vi "Dashboard Main.vi"() -> ()   [LabVIEW 2012]
uses:
  <vilib>/Rock Robotics/WPI/Camera/WPI_CameraWhite Balance Values.ctl
  <vilib>/event_ctls.llb/eventvkey.ctl
  <vilib>/Utility/config.llb/Read Key (String).vi
  <vilib>/Utility/config.llb/Read Key (I32).vi
  <vilib>/Utility/config.llb/Write Key (String).vi
  <vilib>/Utility/config.llb/Write Key (I32).vi
  globals/Angle.vi
  <vilib>/Utility/config.llb/NI_LVConfig.lvlib
  AutonomousSelector.lvlib
  <vilib>/FTP/NI_FTP.lvlib
panel:
  in  "Tab Control":enum32{"Main", "Diagnostic"}(tab)
  in  "Viewer":enum32{"Camera", "Variables", "Files"}(tab)
  in  "Camera Settings":T1={"Frate Rate"=30, "Compression"=30, "Size"=1} {"Frate Rate" scale=1.0..30.0; "Size" items=["640x480", "320x240", "160x120"]}
  out "Mbps":dbl format="%#.1g"
  in  "DB Camera Config":bool
  out "Mbps":bool
  out "fps":dbl format="%#.1g"
  out "Image Error Message":string="Timeout in Camera Communications"
  out "Low Camera Image":T2(plugin-control) caption="Camera Image"
  out "High Camera Image":T2(plugin-control) caption="Camera Image"
  out "Tree":string(tree)
  in  "working directory":path=path "C:/BB/2013/Programming/Beachbot2013Dashboard"
  out "standard output":string
  in  "Transfer CSV to cRIO":bool
  in  "Transfer INI From cRIO":bool
  in  "Dashboard Tab":T3(tab)
  in  "LEDEnable":bool
  out "Battery Value":dbl(slide) scale=0.0..14.0 scale format="%#_2e"
  out "Battery":sgl(graph)
  out "Robot IP":string
  in  "Autonomous Mode":u16(ring)
  in  "Number":dbl caption="rightDriveP"
  in  "Preferences Tree":string(tree)
  in  "Save":bool
  in  "On/Off":bool caption="~S A V E~"
  in  "String":string caption="Strings"
  in  "Slider":dbl(slide) scale=0.0..100.0 scale format="%#_3g"
  in  "What is this?":bool
  in  "Test Name":u16(ring) items=["Select the test to run...", "Example Test", "-------------------------------", "List of tests is built in robot code.", "Replace with your own automated tests."]
  in  "Test Tree":string(tree)
  in  "Motor":cluster{"Value":dbl, "Enable":bool} {"Value" scale=-1.0..1.0 scale format="%#_3g"}
  out "Progress":T4 {"Test Progress" scale=0.0..100.0}
  in  "Rev/Fwd":cluster{"Forward":bool, "Reverse":bool}
  in  "Ring":u16(ring) items=["Auto", "Fixed indoor", "Fixed outdoor 1", "Fixed outdoor 2", "Fixed fluorescent 1", "Fixed fluorescent 2", "Hold current"]
  in  "Listbox":i32(listbox)
  out "Camera Image Diag":T2(plugin-control) caption="Camera Image"
  out "High Camera IP":string
  out "Low Camera IP":string
  out "Target Info":T5(array[cluster]) {"Center Position"."X" format="%#_3g"; "Center Position"."Y" format="%#_3g"}
  in  "Camera view angle":dbl[](array[numeric])=[48.0, 43.5]
  out "Processed Image":T2(plugin-control)
  in  "High Dilate_its":i32=5
  in  "High Erode_its":i32=5
  in  "High Brightness":i32=50
  in  "Low Dilate_its":i32=8
  in  "Low Erode_its":i32=7
  in  "Low Brightness":i32=50
  in  "Camera\nSelect H/L":bool=TRUE
  out "Mode":T6(ring)=enum."Auto Disabled"
  # "Robot IP:"
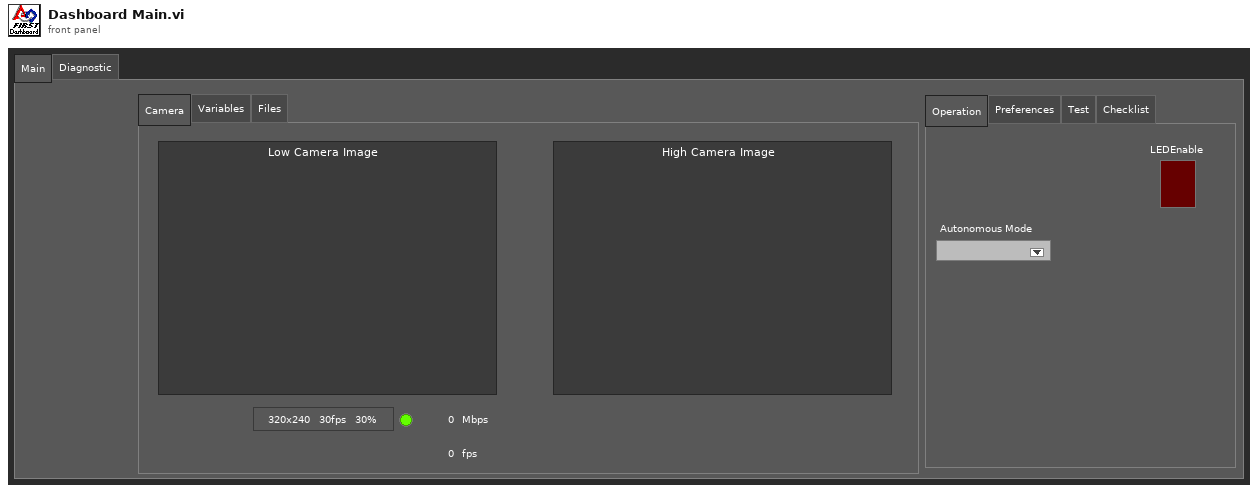
[diagram p1: front panel]
types:
  T1 = cluster{"Frate Rate":i32, "Compression":i32, "Size":u16}
  T2 = typedef "IMAQ Image.ctl" = refnum<image>
  T3 = enum32{"Operation", "Preferences", "Test", "Checklist"}
  T4 = cluster{"Test Progress":u8, "Test Progress Text":string}
  T5 = cluster{"Center Position":cluster{"X":dbl, "Y":dbl}, "Distance":dbl, "targetType":enum16{"Center", "Side", "Vertical"}}[]
  T6 = enum8{"Tele-Op Disabled", "Tele-Op Enabled", "Auto Disabled", "Auto Enabled", "Test Disabled", "Test Enabled", ""}
  T7 = typedef "Image Type" = u32
  T8 = typedef "WPI_CameraWhite Balance Values.ctl" = enum16{"Auto", "Fixed indoor", "Fixed outdoor 1", "Fixed outdoor 2", "Fixed fluorescent 1", "Fixed fluorescent 2", "Hold current"}
  T9 = typedef "SkeletonTrackState.ctl" = enum32{"NotTracked", "PositionOnly", "Tracked"}
  T10 = cluster{"TrackingState":u8[], "Position":cluster{"x":sgl, "y":sgl, "z":sgl}, cluster{"x":sgl, "y":sgl, "z":sgl, sgl}[], "TrackState":T9}
  T11 = cluster{cluster{"ScaledToPercentRange":dbl, "ScaledToPercentRange":dbl, "ScaledToPercentRange":dbl}, cluster{bool, bool, bool}}[]
  T12 = cluster{cluster{"ScaledToPercentRange":dbl, "ScaledToPercentRange":dbl, "ScaledToPercentRange":dbl}, cluster{bool, bool, bool}}
  T13 = typedef "LVRectTypeDef.ctl" = cluster{"Left":i16, "Top":i16, "Right":i16, "Bottom":i16}
  T14 = cluster{"Competition mode":bool, "Robot Link":bool, "Autonomous":bool, "Enabled":bool, "E-Stop":bool, "Simulated":bool, "TestMode":bool, "Docked Window":bool}
  T15 = typedef "NI_LVConfig.lvlib/Config Data RefNum.ctl" = refnum<k1>
  T16 = typedef "WPI_CameraDevRef.ctl" = cluster{"Camera Address":string, "CameraStatus":errorcluster, "Acquire Image Notifier":refnum<notifier>}
  T17 = typedef "eventvkey.ctl" = enum16{"ASCII", "Enter", "Return", "Shift", "Ctrl", "Alt", "Cmd", "Opt", "Caps", "NumLock", "Clear", "Break", "Up", "Down", "Left", "Right", "Insert", "Delete", "Home", "End", "PageUp", "PageDown", "Escape", "Help", "Pause", "ScrollLock", "F1", "F2", "F3", "F4", "F5", "F6", "F7", "F8", "F9", "F10", "F11", "F12", "F13", "F14", "F15", "F16", "F17", "F18", "F19", "F20", "F21", "F22", "F23", "F24", "Play", "VolumeUp", "VolumeDown", "Mute", "Two Byte Char"}
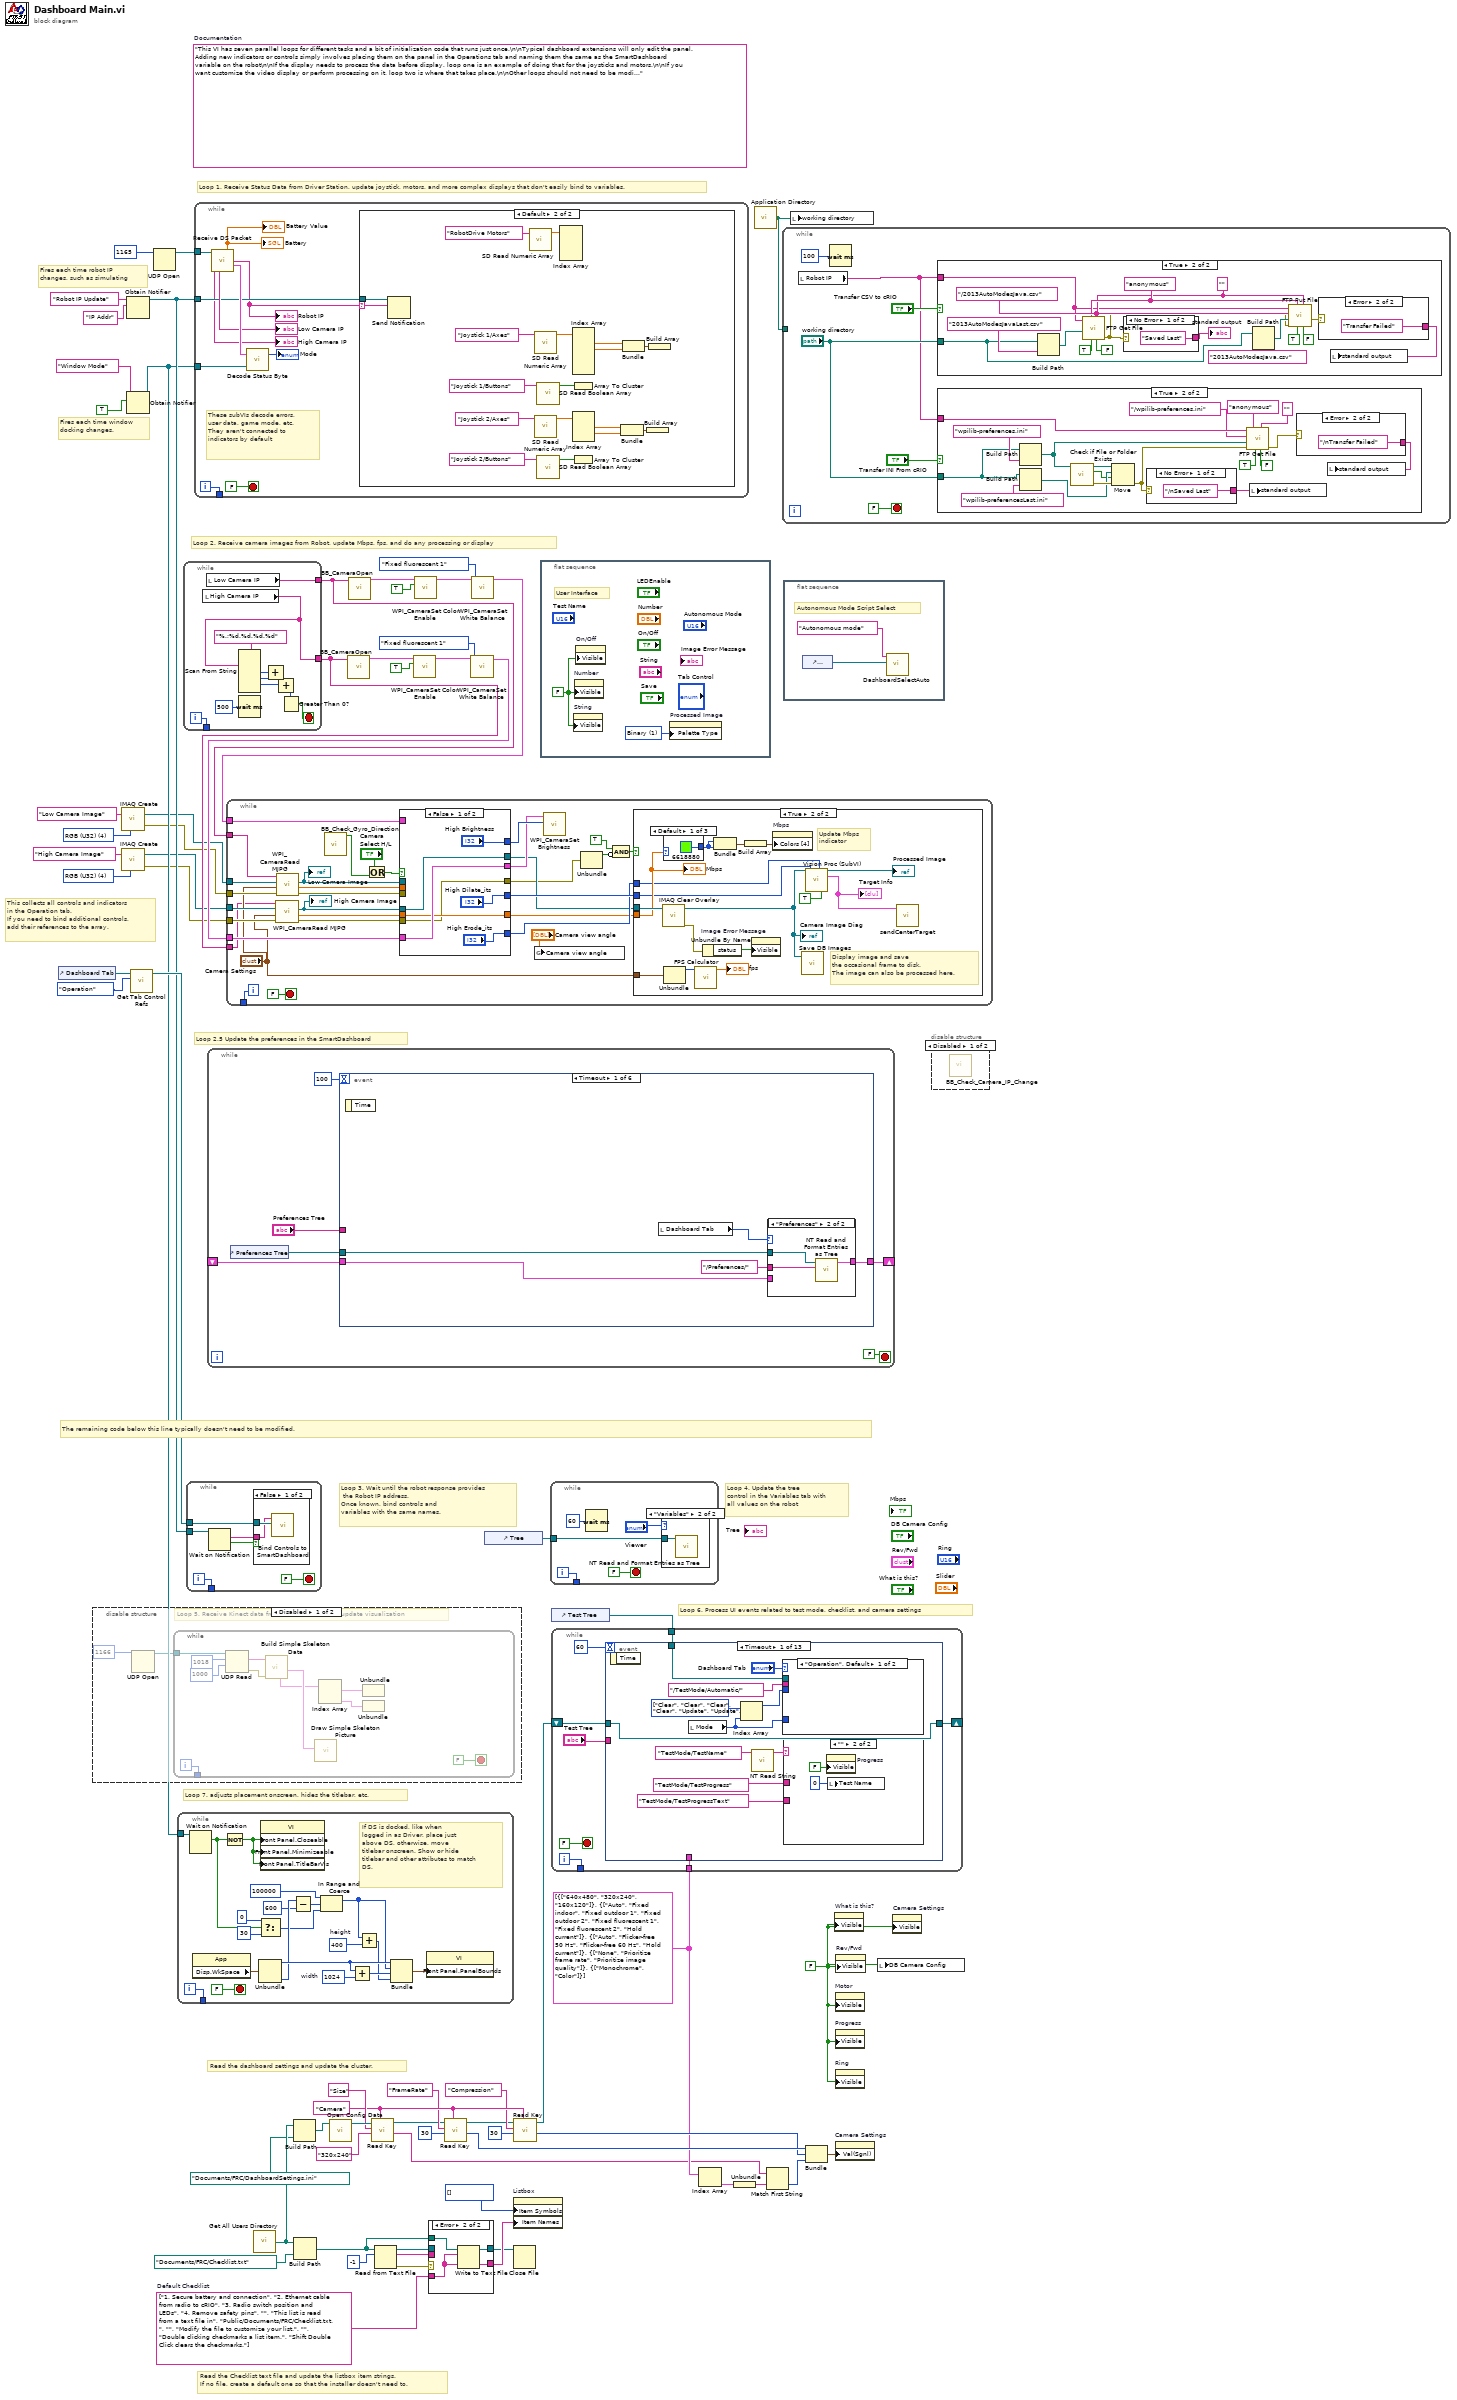
[diagram p0: block diagram]
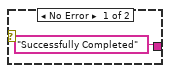
[diagram p3: hidden frame]
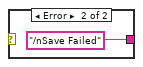
[diagram p4: hidden frame]
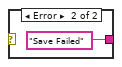
[diagram p6: hidden frame]
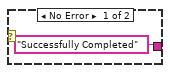
[diagram p7: hidden frame]
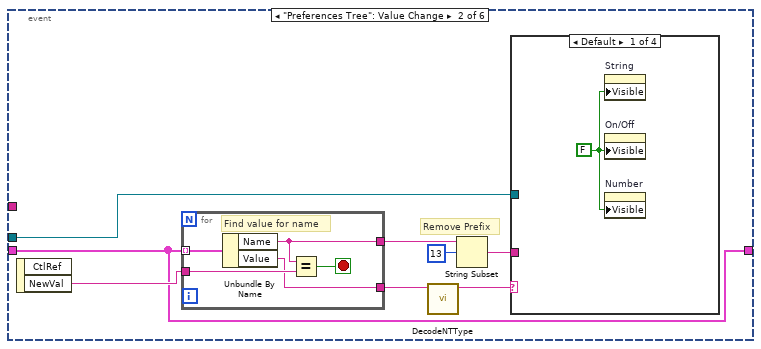
[diagram p10: hidden frame]
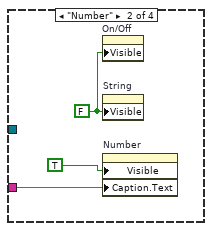
[diagram p11: hidden frame]
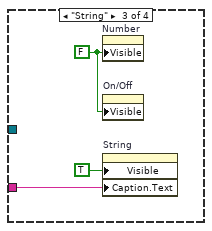
[diagram p12: hidden frame]
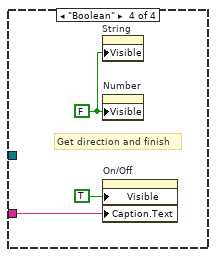
[diagram p13: hidden frame]
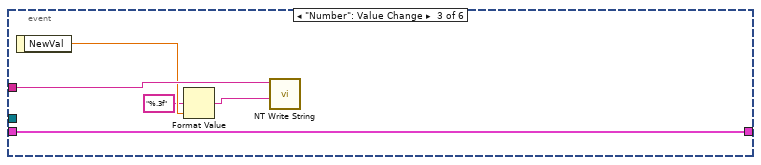
[diagram p14: hidden frame]
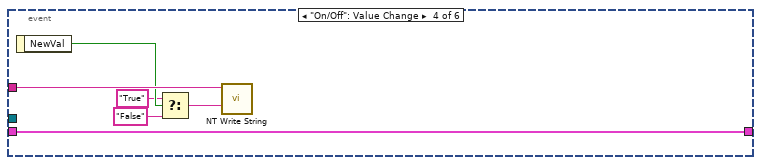
[diagram p15: hidden frame]
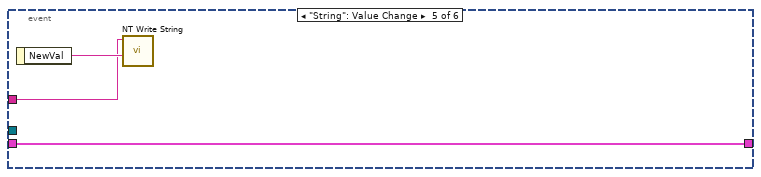
[diagram p16: hidden frame]
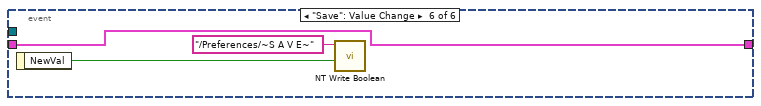
[diagram p17: hidden frame]
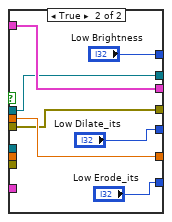
[diagram p20: hidden frame]
diagram:
  w7 = T7 4 items=["Grayscale (U8)", "Grayscale (I16)", "Grayscale (SGL)", "Complex (CSG)", "RGB (U32)", "HSL (U32)", "RGB (U64)"] ("Image Type")
  w8 = T7 4 items=["Grayscale (U8)", "Grayscale (I16)", "Grayscale (SGL)", "Complex (CSG)", "RGB (U32)", "HSL (U32)", "RGB (U64)"] ("Image Type")
  w42 = "Camera"
  w34 = cluster{string[]}[] [{["640x480", "320x240", "160x120"]}, {["Auto", "Fixed indoor", "Fixed outdoor 1", "Fixed outdoor 2", "Fixed fluorescent 1", "Fixed fluorescent 2", "Hold current"]}, {["Auto", "Flicker-free 50 Hz", "Flicker-free 60 Hz", "Hold current"]}, {["None", "Prioritize frame rate", "Prioritize image quality"]}, {["Monochrome", "Color"]}]
  w50 = string[] ["1. Secure battery and connection", "2. Ethernet cable from radio to cRIO", "3. Radio switch position and LEDs", "4. Remove safety pins", "", "This list is read from a text file in", "Public/Documents/FRC/Checklist.txt.", "", "Modify the file to customize your list.", "", "Double clicking checkmarks a list item.", "Shift Double Click clears the checkmarks."]  # Default Checklist
  w48 = FALSE ("Visible")
  (unwired) "This VI has seven parallel loops for different tasks and a bit of initialization code that runs just once.\n\nTypical dashboard extensions will only edit the panel. Adding new indicators or controls simply involves placing them on the panel in the Operations tab and naming them the same as the SmartDashboard variable on the robot\n\nIf the display needs to process the data before display, loop one is an example of doing that for the joysticks and motors.\n\nIf you want customize the video display or perform processing on it, loop two is where that takes place.\n\nOther loops should not need to be modified. They are pretty standard, and document the task they perform."  # Documentation
  # "Loop 2.5 Update the preferences in the SmartDashboard"
  # "Fires each time robot IP\nchanges, such as simulating"
  # "Fires each time window\ndocking changes."
  # "Read the Checklist text file and update the listbox item strings.\nIf no file, create a default one so that the installer doesn't need to."
  # "This collects all controls and indicators\nin the Operation tab.\nIf you need to bind additional controls,\nadd their references to the array."
  # "The remaining code below this line typically doesn't need to be modified."
  # "Loop 6. Process UI events related to test mode, checklist, and camera settings"
  # "Read the dashboard settings and update the cluster."
  # "Loop 4. Update the tree\ncontrol in the Variables tab with\nall values on the robot"
  # "Loop 3. Wait until the robot response provides\n the Robot IP address.\nOnce known, bind controls and\nvariables with the same names."
  # "Loop 7. adjusts placement onscreen, hides the titlebar, etc."
  # "Loop 1. Receive Status Data from Driver Station, update joystick, motors, and more complex displays that don't easily bind to variables."
  # "Loop 2. Receive camera images from Robot, update Mbps, fps, and do any processing or display"
  n1 = control-ref of="Dashboard Tab"() -> (w64:refnum<vi>)
  n2 = disable-structure shown="Disabled" {
    frame Disabled {
      # "Loop 5. Receive Kinect data from Driver Station and update visualization"
      n3 = UDP Open(11:u16 1166 ("port")) -> (port=w68:refnum<k16>)  [unwired: 2 in, 4 out]
      n4 = while {
        tunnel: w68 -> [w78]
        tunnel: [w71] -> _
        i -> [w71]
        stop <- FALSE stop-if-true
        n5 = UDP Read(connection ID=w78, max size (548)=1018 ("bytes to read"), timeout ms (25000)=1000) -> (data out=w76:string, error out=w70:errorcluster)  [unwired: 1 in, 3 out]
        n6 = call "Build Simple Skeleton Data.vi"("error in (no error)"=w70, "data in"=w76) -> ("Skeleton Data"=w77:T10, "Simple Joystick Info"=w74:T11)  [unwired: 5 in, 3 out]
        n7 = call "Draw Simple Skeleton Picture.vi"("Simple Skeleton"=w77) -> ()  [unwired: 10 in, 1 out]
        n8 = Index Array(array=w74) -> (element #1=w73:T12, element #2=w72:T12)  [unwired: 2 in]
        n9 = Unbundle(w73) -> ()  [unwired: 2 out]
        n10 = Unbundle(w72) -> ()  [unwired: 2 out]
      }
    }
    frame Enabled {
    }
  }
  n11 = call "IMAQ Create"("Image Name"="Low Camera Image", "Image Type"=w7) -> ("New Image"=w2:T2, "error out"=w3:errorcluster)  [unwired: 2 in, 1 out]
  n12 = call "IMAQ Create"("Image Name"="High Camera Image", "Image Type"=w8) -> ("New Image"=w4:T2, "error out"=w5:errorcluster)  [unwired: 2 in, 1 out]
  n13 = Obtain Notifier(name (unnamed)="Robot IP Update", notification data type="IP Addr" ("name (unnamed)")) -> (notifier out=w61:refnum<notifier>)  [unwired: 2 in, 2 out]
  n14 = Obtain Notifier(name (unnamed)="Window Mode", notification data type=TRUE) -> (notifier out=w54:refnum<notifier>)  [unwired: 2 in, 2 out]
  n15 = call <vilib>:"Get Tab Control Refs.vi"("Page Index"=enum32{"Operation", "Test"}."Operation" ("Dashboard Tab"), "TabControl in"=w64) -> ("ControlsOnPage"=w65:refnum<vi>[])  [unwired: 9 in]
  n16 = UDP Open(11:u16 1165 ("port")) -> (port=w66:refnum<k16>)  [unwired: 2 in, 4 out]
  n17 = while {
    tunnel: w54 -> [w99]
    tunnel: [w97] -> _
    i -> [w97]
    stop <- FALSE stop-if-true
    w89 = 1024  # width
    w92 = 400  # height
    # "If DS is docked, like when\nlogged in as Driver, place just\nabove DS, otherwise, move\ntitlebar onscreen. Show or hide\ntitlebar and other attributes to match\nDS."
    n18 = Wait on Notification(notifier=w99) -> (notification=w84:bool)  [unwired: 3 in, 3 out]
    n19 = property class="App"() -> ("Disp.WkSpace"=w95:T13)  [unwired: 2 in, 2 out]
    n20 = Not(x=w84) -> (.not. x?=w98:bool)
    n21 = Unbundle(w95) -> ("Left"=w93:i16, "Bottom"=w90:i16)  [unwired: 2 out]
    n22 = Select(t=0, s=w84, f=30) -> (s? t:f=w83:i32)
    n23 = property class="VI"("Front Panel.Closeable"=w98, "Front Panel.Minimizeable"=w98, "Front Panel.TitleBarVis"=w98) -> ()  [unwired: 2 in, 2 out]
    n24 = Subtract(x=w90, y=600) -> (x-y=w87:i32)
    n25 = In Range and Coerce(upper limit=100000, x=w87, lower limit=w83) -> (coerced(x)=w81:i32)  [unwired: 1 out]
    n26 = Add(x=w93, y=w89) -> (x+y=w94:i32)
    n27 = Add(x=w81, y=w92) -> (x+y=w91:i32)
    n28 = Bundle("Left"=w93, w81, w94, w91) -> (w96:cluster{"Left":i16, i32, i32, i32})  [unwired: 1 out]
    n29 = property class="VI"("Front Panel.PanelBounds"=w96) -> ()  [unwired: 2 in, 2 out]
  }
  n30 = while {
    tunnel: [w111] -> w11
    tunnel: [w104] -> w10
    tunnel: [w102] -> _
    i -> [w102]
    stop <- w103 stop-if-true
    n31 = local read "High Camera IP"() -> (w104:string)
    n32 = local read "Low Camera IP"() -> (w111:string)
    n33 = Scan From String(format string="%.;%d.%d.%d.%d", input string=w104) -> (output 1=w108:i32, output 2=w109:i32, output 3=w106:i32)  [unwired: 2 in, 8 out]
    n34 = Wait (ms)(milliseconds to wait=u32 500) -> ()  [unwired: 1 out]
    n35 = Add(x=w108, y=w109) -> (x+y=w107:i32)
    n36 = Add(x=w107, y=w106) -> (x+y=w105:i32)
    n37 = Greater Than 0?(x=w105) -> (x > 0?=w103:bool)
  }
  n38 = while {
    tunnel: w65 -> [w117]
    tunnel: w61 -> [w114]
    tunnel: [w112] -> _
    i -> [w112]
    stop <- FALSE stop-if-true
    n39 = Wait on Notification(notifier=w114) -> (notification=w113:string, timed out?=w115:bool)  [unwired: 3 in, 2 out]
    n40 = case shown="False" w115 {
      tunnel: w117 -> [w119 _]
      tunnel: w113 -> [w118 _]
      frame False {
        n41 = call <vilib>:"Bind Controls to SmartDashboard.vi"("Bound Control Refs"=w119, "Server IP Address"=w118) -> ()  [unwired: 10 in]
      }
      frame True {
      }
    }
  }
  n42 = while {
    tunnel: w66 -> [w128]
    tunnel: w61 -> [w122]
    tunnel: w54 -> [w126]
    tunnel: [w123] -> _
    i -> [w123]
    stop <- FALSE stop-if-true
    # "These subVIs decode errors, user data, game mode, etc.\nThey aren't connected to indicators by default"
    n43 = call "Receive DS Packet.vi"("Recv Socket"=w128) -> ("Battery"=→"Battery" →"Battery Value":sgl, "Robot IP Address"=w121:string, "Status"=w129:T14, "High Camera IP Address"=→"High Camera IP":string, "Low Camera IP Address"=→"Low Camera IP":string)  [unwired: 1 in, 9 out]
    "Robot IP" <- w121
    n44 = call "Decode Status Byte.vi"("Window Mode Notifier"=w126, "Status"=w129) -> ("Mode"=→"Mode":T6)  [unwired: 1 out]
    n45 = case shown="Default" w121 {
      selector: w121 -> [_ w131]
      tunnel: w122 -> [_ w132]
      frame "0.0.0.0" {
        # "Robot not responding, don't poll the variables"
      }
      frame Default {
        n46 = Send Notification(notification=w131, notifier=w132) -> ()  [unwired: 1 in, 2 out]
        n47 = call <vilib>:"SD Read Numeric Array.vi"("Name"="RobotDrive Motors") -> ("Numeric Array"=w145:dbl[])  [unwired: 8 in, 2 out]
        n48 = call <vilib>:"SD Read Numeric Array.vi"("Name"="Joystick 1/Axes") -> ("Numeric Array"=w143:dbl[])  [unwired: 8 in, 2 out]
        n49 = call <vilib>:"SD Read Numeric Array.vi"("Name"="Joystick 2/Axes") -> ("Numeric Array"=w139:dbl[])  [unwired: 8 in, 2 out]
        n50 = call <vilib>:"SD Read Boolean Array.vi"("Name"="Joystick 1/Buttons") -> ("Boolean Array"=w144:bool[])  [unwired: 8 in, 2 out]
        n51 = call <vilib>:"SD Read Boolean Array.vi"("Name"="Joystick 2/Buttons") -> ("Boolean Array"=w138:bool[])  [unwired: 8 in, 2 out]
        n52 = Index Array(array=w145) -> ()  [unwired: 4 in, 4 out]
        n53 = Array To Cluster(array=w144) -> ()  [unwired: 1 out]
        n54 = Array To Cluster(array=w138) -> ()  [unwired: 1 out]
        n55 = Index Array(array=w143) -> (element #1=w141:dbl, element #2=w142:dbl)  [unwired: 6 in, 4 out]
        n56 = Index Array(array=w139) -> (element #1=w134:dbl, element #2=w133:dbl)  [unwired: 3 in, 1 out]
        n57 = Bundle("Numeric"=w134, "Numeric"=w133) -> (w135:cluster{"Numeric":dbl, "Numeric":dbl})  [unwired: 1 in]
        n58 = Bundle("Numeric"=w141, "Numeric"=w142) -> (w140:cluster{"Numeric":dbl, "Numeric":dbl})  [unwired: 1 in]
        n59 = Build Array(w135) -> ()  [unwired: 1 out]
        n60 = Build Array(w140) -> ()  [unwired: 1 out]
      }
    }
  }
  n61 = while {
    shift-right: [w150] -> _
    shift-left: _ -> [w149]
    stop <- FALSE stop-if-true
    n62 = control-ref of="Preferences Tree"() -> (w152:refnum<vi>)
    n63 = event shown="[0] Timeout" {
      selector: _ -> [_ _ _ _ _ _]
      dyn-events: _ -> [_ _ _ _ _ _]
      timeout: u32 100 ("milliseconds to wait") -> [_ _ _ _ _ _]
      tunnel: w152 -> [w157 w170 _ _ _ _]
      tunnel: "Preferences Tree" -> [_ _ w191 w197 w199 _]
      tunnel: [w158 w164 w190 w196 w198 w201] -> w150
      tunnel: w149 -> [w156 w164 w190 w196 w198 w201]
      event Timeout {
        n64 = event-data() -> ()  [unwired: 1 in, 1 out]
        n65 = local read "Dashboard Tab"() -> (w155:T3)
        n66 = case shown="\"Preferences\"" w155 {
          tunnel: w157 -> [_ w163]
          tunnel: "/Preferences/" ("Name Pattern") -> [_ w162]
          tunnel: [w160 w161] -> w158
          tunnel: w156 -> [w160 _]
          frame "Operation", Default {
          }
          frame "Preferences" {
            n67 = call <vilib>:"NT Read and Format Entries as Tree.vi"("Name Pattern"=w162, "Tree Refnum"=w163) -> ("Formatted Strings"=w161:cluster{"Name":string, "Value":string}[])  [unwired: 8 in, 1 out]
          }
        }
      }
      event "Preferences Tree": Value Change {
        # "Remove Prefix"
        n68 = event-data() -> ("NewVal"=w168:string)  [unwired: 1 in, 1 out]
        n69 = for {
          tunnel: w164 -> [w176] mode=indexing
          tunnel: w168 -> [w175]
          tunnel: [w173] -> w169
          tunnel: [w172] -> w167
          stop <- w174 stop-if-true
          # "Find value for name"
          n70 = Unbundle By Name(w176) -> ("Name"=w172:string, "Value"=w173:string)
          n71 = Equal?(x=w172, y=w175) -> (x = y?=w174:bool)
        }
        n72 = call "DecodeNTType.vi"("string"=w169) -> ("type"=w171:string)  [unwired: 7 in, 3 out]
        n73 = String Subset(string=w167, offset (0)=13) -> (substring=w166:string)  [unwired: 1 in]
        n74 = case shown="Default" w171 {
          tunnel: w170 -> [_ _ _ _]
          tunnel: w166 -> [_ w178 w181 w185]
          frame Default {
            w177 = FALSE ("Visible")
            n75 = property on="String" class="Str"("Visible"=w177) -> ()  [unwired: 2 in, 2 out]
            n76 = property on="On/Off" class="Bool (strict)"("Visible"=w177) -> ()  [unwired: 2 in, 2 out]
            n77 = property on="Number" class="DigNum (strict)"("Visible"=w177) -> ()  [unwired: 2 in, 2 out]
          }
          frame "Number" {
            w179 = FALSE ("Visible")
            n78 = property on="On/Off" class="Bool (strict)"("Visible"=w179) -> ()  [unwired: 2 in, 2 out]
            n79 = property on="String" class="Str"("Visible"=w179) -> ()  [unwired: 2 in, 2 out]
            n80 = property on="Number" class="DigNum (strict)"("Visible"=TRUE, "Caption.Text"=w178) -> ()  [unwired: 2 in, 2 out]
          }
          frame "String" {
            w182 = FALSE ("Visible")
            n81 = property on="Number" class="DigNum (strict)"("Visible"=w182) -> ()  [unwired: 2 in, 2 out]
            n82 = property on="On/Off" class="Bool (strict)"("Visible"=w182) -> ()  [unwired: 2 in, 2 out]
            n83 = property on="String" class="Str"("Visible"=TRUE, "Caption.Text"=w181) -> ()  [unwired: 2 in, 2 out]
          }
          frame "Boolean" {
            w184 = FALSE ("Visible")
            # "Get direction and finish"
            n84 = property on="String" class="Str"("Visible"=w184) -> ()  [unwired: 2 in, 2 out]
            n85 = property on="Number" class="DigNum (strict)"("Visible"=w184) -> ()  [unwired: 2 in, 2 out]
            n86 = property on="On/Off" class="Bool (strict)"("Visible"=TRUE, "Caption.Text"=w185) -> ()  [unwired: 2 in, 2 out]
          }
        }
      }
      event "Number": Value Change {
        n87 = event-data() -> ("NewVal"=w189:dbl)  [unwired: 1 in]
        n88 = Format Value(format string="%.3f", value (0)=w189) -> (output string=w187:string)  [unwired: 1 in]
        n89 = call <vilib>:"NT Write String.vi"("String"=w187, "Name"=w191) -> ()  [unwired: 9 in, 1 out]
      }
      event "On/Off": Value Change {
        n90 = event-data() -> ("NewVal"=w195:bool)  [unwired: 1 in]
        n91 = Select(t="True", s=w195, f="False") -> (s? t:f=w192:string)
        n92 = call <vilib>:"NT Write String.vi"("String"=w192, "Name"=w197) -> ()  [unwired: 9 in, 1 out]
      }
      event "String": Value Change {
        n93 = event-data() -> ("NewVal"=w200:string)  [unwired: 1 in]
        n94 = call <vilib>:"NT Write String.vi"("String"=w200, "Name"=w199) -> ()  [unwired: 9 in, 1 out]
      }
      event "Save": Value Change {
        n95 = event-data() -> ("NewVal"=w203:bool)  [unwired: 1 in]
        n96 = call <vilib>:"NT Write Boolean.vi"("Boolean"=w203, "Name"="/Preferences/~S A V E~") -> ()  [unwired: 9 in, 1 out]
      }
    }
  }
  n97 = call "Get All Users Directory.vi"() -> ("All User Path"=w47:path)
  n98 = Build Path(base path=w47, name or relative path=path "Documents/FRC/DashboardSettings.ini") -> (appended path=w46:path)
  n99 = Build Path(base path=w47, name or relative path=path "Documents/FRC/Checklist.txt") -> (appended path=w51:path)
  n100 = call <vilib>:"Open Config Data.vi"("configuration file path"=w46) -> ("refnum"=w45:T15)  [unwired: 8 in, 2 out]
  n101 = call "BB_CameraOpen.vi"("Camera Address"=w10) -> ("CameraDevRef"=w17:T16)  [unwired: 9 in, 1 out]
  n102 = call "BB_CameraOpen.vi"("Camera Address"=w11) -> ("CameraDevRef"=w21:T16)  [unwired: 9 in, 1 out]
  n103 = call-poly <vilib>:"Read Key.vi"("section"=w42, "default value"="320x240", "key"="Size", "refnum"=w45) -> ("value"=w32:string, "refnum out"=w27:T15)  [unwired: 2 in, 4 out]
  n104 = Read from Text File(file (use dialog)=w51, count=-1 ("timeout ms (25000)")) -> (refnum out=w29:refnum<file>, text=w52:string[], error out=w53:errorcluster)  [unwired: 2 in, 1 out]
  n105 = call <vilib>:"WPI_CameraSet Color Enable.vi"("Color Enabled"=TRUE, "CameraDevRef"=w17) -> ("CameraDevRef Out"=w15:T16)  [unwired: 8 in, 1 out]
  n106 = call <vilib>:"WPI_CameraSet Color Enable.vi"("Color Enabled"=TRUE, "CameraDevRef"=w21) -> ("CameraDevRef Out"=w19:T16)  [unwired: 8 in, 1 out]
  n107 = case shown="Error" w53 {
    tunnel: w52 -> [w205 _]
    tunnel: [w205 w207] -> w49
    tunnel: w50 -> [_ w207]
    tunnel: w51 -> [_ w208]
    tunnel: [w204 w206] -> w28
    tunnel: w29 -> [w204 _]
    frame No Error {
    }
    frame Error {
      n108 = Write to Text File(file (use dialog)=w208, text=w207) -> (refnum out=w206:refnum<file>)  [unwired: 2 in, 2 out]
    }
  }
  n109 = call-poly <vilib>:"Read Key.vi"("section"=w42, "default value"=30, "key"="FrameRate", "refnum"=w27) -> ("value"=w37:i32, "refnum out"=w26:T15)  [unwired: 1 in, 5 out]
  n110 = call <vilib>:"WPI_CameraSet White Balance.vi"("White Balance"=WPI_CameraWhite_Balance_Values."Fixed fluorescent 1", "CameraDevRef"=w15) -> ("CameraDevRef Out"=w13:T16)  [unwired: 8 in, 1 out]
  n111 = call <vilib>:"WPI_CameraSet White Balance.vi"("White Balance"=WPI_CameraWhite_Balance_Values."Fixed fluorescent 1", "CameraDevRef"=w19) -> ("CameraDevRef Out"=w12:T16)  [unwired: 8 in, 1 out]
  n112 = while {
    tunnel: [w238] -> _
    tunnel: w13 -> [w230]
    tunnel: w12 -> [w231]
    tunnel: w10 -> [w212]
    tunnel: w11 -> [w213]
    tunnel: w5 -> [w224]
    tunnel: w4 -> [w223]
    tunnel: w3 -> [w222]
    tunnel: w2 -> [w220]
    i -> [w238]
    stop <- FALSE stop-if-true
    n113 = call <vilib>:"WPI_CameraRead MJPG.vi"("error in"=w224, "Camera Settings"="Camera Settings", "Image"=w223, "address"=w212) -> ("error out"=w216:errorcluster, "Bandwidth (kbps)"=w215:dbl, "Image Out"=w214:T2)  [unwired: 5 in]
    "High Camera Image" <- w214
    n114 = call <vilib>:"WPI_CameraRead MJPG.vi"("error in"=w222, "Camera Settings"="Camera Settings", "Image"=w220, "address"=w213) -> ("error out"=w218:errorcluster, "Bandwidth (kbps)"=w219:dbl, "Image Out"=w217:T2)  [unwired: 5 in]
    "Low Camera Image" <- w217
    n115 = call "BB_Check_Gyro_Direction.vi"() -> ("chgDirection"=w226:bool)  [unwired: 11 in]
    n116 = Or(x="Camera\nSelect H/L", y=w226) -> (x .or. y?=w227:bool)
    n117 = case shown="False" w227 {
      tunnel: w231 -> [_ w253]
      tunnel: [w243 w253] -> w229
      tunnel: ["High Dilate_its" "Low Dilate_its"] -> w233
      tunnel: ["High Erode_its" "Low Erode_its"] -> w232
      tunnel: ["High Brightness" "Low Brightness"] -> w234
      tunnel: w230 -> [w243 _]
      tunnel: [w242 w249] -> w210
      tunnel: w219 -> [_ w248]
      tunnel: w218 -> [_ w247]
      tunnel: w217 -> [_ w249]
      tunnel: w216 -> [w240 _]
      tunnel: w215 -> [w241 _]
      tunnel: w214 -> [w242 _]
      tunnel: [w241 w248] -> w211
      tunnel: [w240 w247] -> w209
      frame False {
      }
      frame True {
      }
    }
    n118 = global write "Angle.vi" "Camera view angle"("Camera view angle") -> ()
    n119 = call <vilib>:"WPI_CameraSet Brightness.vi"("Brightness"=w234, "CameraDevRef"=w229) -> ()  [unwired: 8 in, 2 out]
    n120 = Unbundle(w209) -> ("status"=w237:bool)  [unwired: 2 out]
    n121 = Compound Arithmetic op=AND(TRUE, invert w237) -> (w236:bool)
    n122 = case shown="True" w236 {
      tunnel: "Camera Settings" -> [_ w262]
      tunnel: w210 -> [_ w265]
      tunnel: w211 -> [_ w264]
      tunnel: w233 -> [_ w259]
      tunnel: w232 -> [_ w258]
      frame False {
        # "Sleep for 500ms"
        n123 = Wait Until Next ms Multiple(millisecond multiple=u32 500) -> ()  [unwired: 1 out]
      }
      frame True {
        # "Display image and save\nthe occasional frame to disk.\nThe image can also be processed here."
        # "Update Mbps\nindicator"
        n124 = call "IMAQ Clear Overlay"("Image"=w265) -> ("error out"=w269:errorcluster, "Image Out"=w257:T2)  [unwired: 2 in, 7 out]
        "Camera Image Diag" <- w257
        n125 = case shown="Default" w264 {
          tunnel: [u32 6618880 ("Color Box") u32 16776722 ("Color Box") u32 16716800 ("Color Box")] -> w266
          frame Default {
          }
          frame 4, 5 {
          }
          frame 6.. {
          }
        }
        n126 = Unbundle(w262) -> ("Frate Rate"=w261:i32)  [unwired: 2 out]
        n127 = call "FPS Calculator.vi"("Average Count"=w261) -> ("fps"=→"fps":dbl)  [unwired: 10 in]
        n128 = Unbundle By Name(w269) -> ("status"=w270:bool)
        n129 = Bundle("Color Box"=w266, "Color Box"=w266) -> (w268:cluster{"Color Box":u32, "Color Box":u32})  [unwired: 1 out]
        n130 = Build Array(w268) -> (w267:cluster{"Color Box":u32, "Color Box":u32}[])
        n131 = property on="Image Error Message" class="Str"("Visible"=w270) -> ()  [unwired: 2 in, 2 out]
        n132 = property on="Mbps" class="Bool (strict)"("Colors [4]"=w267) -> ()  [unwired: 2 in, 2 out]
        n133 = call "Save DB Images.vi"("Image"=w257) -> ()  [unwired: 2 in, 1 out]
        n134 = call "Vision Proc (SubVI).vi"("Image In"=w257, "Dilate_its"=w259, "Erode_its"=w258, "Annotate"=TRUE) -> ("Processed Image"=→"Processed Image":T2, "Target Info"=w255:T5)  [unwired: 19 in, 3 out]
        "Target Info" <- w255
        n135 = call "sendCenterTarget.vi"("Target Info"=w255) -> ()  [unwired: 11 in]
        "Mbps" <- w264
      }
    }
  }
  n136 = control-ref of="Tree"() -> (w23:refnum<vi>)
  n137 = property on="Listbox" class="LstBox (strict)"("Item Symbols"=i32[] [], "Item Names"=w49) -> ()  [unwired: 2 in, 2 out]
  n138 = Close File(refnum=w28) -> ()  [unwired: 1 in, 2 out]
  n139 = call-poly <vilib>:"Read Key.vi"("section"=w42, "default value"=30, "key"="Compression", "refnum"=w26) -> ("value"=w36:i32, "refnum out"=w24:T15)  [unwired: 1 in, 5 out]
  n140 = flat-sequence {
    frame #0 {
      w274 = FALSE ("Visible")
      w275 = u32 1 items=["Grayscale", "Binary", "Gradient", "Rainbow", "Temperature", "User Defined"] ("Palette:Palette Type")
      # "User Interface"
      n141 = property on="String" class="Str"("Visible"=w274) -> ()  [unwired: 2 in, 2 out]
      n142 = property on="Number" class="DigNum (strict)"("Visible"=w274) -> ()  [unwired: 2 in, 2 out]
      n143 = property on="On/Off" class="Bool (strict)"("Visible"=w274) -> ()  [unwired: 2 in, 2 out]
      n144 = property on="Processed Image" class="ImageControl"("Palette Type"=w275) -> ()  [unwired: 2 in, 2 out]
    }
  }
  n145 = while {
    tunnel: [w277] -> _
    tunnel: w23 -> [w276]
    i -> [w277]
    stop <- FALSE stop-if-true
    n146 = Wait (ms)(milliseconds to wait=u32 60) -> ()  [unwired: 1 out]
    n147 = case shown="\"Variables\"" "Viewer" {
      tunnel: w276 -> [_ w281]
      frame Default {
      }
      frame "Variables" {
        n148 = call <vilib>:"NT Read and Format Entries as Tree.vi"("Tree Refnum"=w281) -> ()  [unwired: 9 in, 2 out]
      }
    }
  }
  n149 = control-ref of="Test Tree"() -> (w22:refnum<vi>)
  n150 = while {
    tunnel: w34 -> [w286]
    shift-right: [w285] -> _
    shift-left: w24 -> [w284]
    tunnel: [w283] -> _
    tunnel: w22 -> [w282]
    i -> [w283]
    stop <- FALSE stop-if-true
    n151 = event shown="[0] Timeout" {
      selector: _ -> [_ _ _ _ _ _ _ _ _ _ _ _ _]
      dyn-events: _ -> [_ _ _ _ _ _ _ _ _ _ _ _ _]
      timeout: u32 60 ("milliseconds to wait") -> [_ _ _ _ _ _ _ _ _ _ _ _ _]
      tunnel: w282 -> [w296 _ _ _ _ _ _ _ _ _ _ _ _]
      tunnel: "Test Tree" -> [_ _ _ _ _ _ _ _ w490 w498 w500 w504 w512]
      tunnel: w286 -> [_ w318 _ _ _ _ w454 w484 _ _ _ _ _]
      tunnel: [w290 w317 _ w420 w428 w440 w453 w477 w489 w496 w499 w503 w511] -> w285
      tunnel: w284 -> [w290 w317 _ w420 w428 w440 w452 w477 w489 w496 w499 w503 w511]
      event Timeout {
        w295 = enum16{"Update", "Clear"}[] [enum."Clear", enum."Clear", enum."Clear", enum."Clear", enum."Update", enum."Update", enum."Clear"] items=["Update", "Clear"]
        n152 = event-data() -> ()  [unwired: 1 in, 1 out]
        n153 = local read "Mode"() -> (w293:T6)
        n154 = Index Array(array=w295, index=w293) -> (element=w294:enum16{"Update", "Clear"})
        n155 = call <vilib>:"NT Read String.vi"("Name"="TestMode/TestName") -> ("String"=w299:string)  [unwired: 9 in, 1 out]
        n156 = case shown="\"Operation\", Default" "Dashboard Tab" {
          tunnel: w296 -> [_ w309]
          tunnel: "/TestMode/Automatic/" ("Name Pattern") -> [_ w308]
          tunnel: w294 -> [_ w307]
          tunnel: w293 -> [_ w305]
          frame "Operation", Default {
          }
          frame "Test" {
            w304 = -2 ("Active Item:Row Number")
            n157 = call <vilib>:"NT Read and Format Entries as Tree.vi"("Operation"=w307, "Name Pattern"=w308, "Tree Refnum"=w309) -> ()  [unwired: 7 in, 2 out]
            n158 = Index Array(array=u32[] [14013909, 14013909, 14013909, 14013909, 14013909, 16777215, 14013909], index=w305) -> (element=w303:u32)
            n159 = property on="Test Tree" class="Tree (strict)"("Active Item Row Number"=w304, "ActiveColNum"=w304, "CellBG"=w303, "Active Item Row Number"=-1 ("Active Item:Row Number"), "CellBG"=u32 5789784 ("Color Box")) -> ()  [unwired: 2 in, 2 out]
          }
        }
        n160 = case shown="\"\"" w299 {
          tunnel: "TestMode/TestProgress" ("Name") -> [w311 _]
          tunnel: "TestMode/TestProgressText" ("Name") -> [w310 _]
          frame Default {
            n161 = call <vilib>:"NT Read Number.vi"("Name"=w311) -> ("Numeric"=w312:dbl)  [unwired: 9 in, 1 out]
            n162 = call <vilib>:"NT Read String.vi"("Name"=w310) -> ("String"=w313:string)  [unwired: 9 in, 1 out]
            n163 = Bundle("Numeric"=w312, "String"=w313) -> (→"Progress":cluster{"Numeric":dbl, "String":string})  [unwired: 1 in]
          }
          frame "" {
            n164 = property on="Progress" class="Clust (strict)"("Visible"=FALSE) -> ()  [unwired: 2 in, 2 out]
            n165 = local write "Test Name"(u16 0) -> ()
          }
        }
      }
      event "Test Tree": Value Change {
        # "Show appropriate\ncontrols"
        n166 = event-data() -> ("CtlRef"=w321:refnum<vi>, "NewVal"=w319:string)  [unwired: 1 in]
        n167 = call <vilib>:"WPI_UtilitiesGetTreeIOName.vi"("NewVal"=w319, "TreeControl in"=w321) -> ("I/O Name"=w322:string)  [unwired: 9 in]
        n168 = case shown="\"Compressor\", \"Digital Out\"" w322 {
          selector: w322 -> [_ w329 _ w347 w356 _]
          tunnel: w319 -> [_ _ w344 w346 _ w363]
          tunnel: w318 -> [_ _ _ _ _ w362]
          frame Default {
            w324 = FALSE ("Visible")
            w323 = FALSE ("Visible")
            n169 = property on="Motor" class="Clust (strict)"("Visible"=w323) -> ()  [unwired: 2 in, 2 out]
            n170 = property on="Ring" class="Ring (strict)"("Visible"=w323) -> ()  [unwired: 2 in, 2 out]
            n171 = property on="Rev/Fwd" class="Clust (strict)"("Visible"=w324) -> ()  [unwired: 2 in, 2 out]
            n172 = property on="What is this?" class="Bool (strict)"("Visible"=w324) -> ()  [unwired: 2 in, 2 out]
            n173 = property on="Slider" class="Slide (strict)"("Visible"=w324) -> ()  [unwired: 2 in, 2 out]
          }
          frame "Motor", "PWM" {
            w330 = FALSE ("Visible")
            n174 = case shown="\"Motor\", Default" w329 {
              tunnel: [1.0 ("Value") -1.0 ("Value")] -> w328
              tunnel: [255.0 ("Value") 1.0 ("Value")] -> w327
              tunnel: [128.0 ("Value") 0.0 ("Value")] -> w326
              tunnel: [64.0 ("Value") 0.5 ("Value")] -> w325
              frame "PWM" {
              }
              frame "Motor", Default {
              }
            }
            n175 = property on="Motor" class="Clust (strict)"("Visible"=TRUE) -> ()  [unwired: 2 in, 2 out]
            n176 = property on="Value" class="Slide (strict)"("Value"=w326, "Scale.Minimum"=w328, "Scale.Maximum"=w327, "Scale.Increment"=w325) -> ()  [unwired: 2 in, 2 out]
            n177 = property on="What is this?" class="Bool (strict)"("Visible"=w330) -> ()  [unwired: 2 in, 2 out]
            n178 = property on="Slider" class="Slide (strict)"("Visible"=w330) -> ()  [unwired: 2 in, 2 out]
            n179 = property on="Ring" class="Ring (strict)"("Visible"=w330) -> ()  [unwired: 2 in, 2 out]
            n180 = property on="Rev/Fwd" class="Clust (strict)"("Visible"=w330) -> ()  [unwired: 2 in, 2 out]
          }
          frame "Servo" {
            w342 = FALSE ("Visible")
            n181 = call <vilib>:"NT Read Number.vi"("Name"=w344) -> ("Numeric"=w343:dbl)  [unwired: 9 in, 1 out]
            n182 = property on="Slider" class="Slide (strict)"("Visible"=TRUE, "Scale.Maximum"=170.0 ("Scale.Range:Maximum")) -> ()  [unwired: 2 in, 2 out]
            n183 = local write "Slider"(w343) -> ()
            n184 = property on="Motor" class="Clust (strict)"("Visible"=w342) -> ()  [unwired: 2 in, 2 out]
            n185 = property on="Rev/Fwd" class="Clust (strict)"("Visible"=w342) -> ()  [unwired: 2 in, 2 out]
            n186 = property on="What is this?" class="Bool (strict)"("Visible"=w342) -> ()  [unwired: 2 in, 2 out]
            n187 = property on="Ring" class="Ring (strict)"("Visible"=w342) -> ()  [unwired: 2 in, 2 out]
          }
          frame "Relay", "Solenoid" {
            w345 = FALSE ("Visible")
            n188 = property on="Motor" class="Clust (strict)"("Visible"=w345) -> ()  [unwired: 2 in, 2 out]
            n189 = property on="Slider" class="Slide (strict)"("Visible"=w345) -> ()  [unwired: 2 in, 2 out]
            n190 = Search and Replace String(input string=w346, search string="/Value  **", replace string="/Direction") -> (result string=w352:string)  [unwired: 5 in, 3 out]
            n191 = property on="Ring" class="Ring (strict)"("Visible"=w345) -> ()  [unwired: 2 in, 2 out]
            n192 = call <vilib>:"NT Read String.vi"("Name"=w352) -> ("String"=w350:string)  [unwired: 9 in, 1 out]
            n193 = Equal?(x="Both directions", y=w350) -> (x = y?=w348:bool)
            n194 = Not(x=w348) -> (.not. x?=w349:bool)
            n195 = property on="Rev/Fwd" class="Clust (strict)"("Visible"=w348) -> ()  [unwired: 2 in, 2 out]
            n196 = property on="What is this?" class="Bool (strict)"("Visible"=w349, "Caption.Text"=w347) -> ()  [unwired: 2 in, 2 out]
          }
          frame "Compressor", "Digital Out" {
            w355 = FALSE ("Visible")
            # "Get direction and finish"
            n197 = property on="Motor" class="Clust (strict)"("Visible"=w355) -> ()  [unwired: 2 in, 2 out]
            n198 = property on="Slider" class="Slide (strict)"("Visible"=w355) -> ()  [unwired: 2 in, 2 out]
            n199 = property on="Ring" class="Ring (strict)"("Visible"=w355) -> ()  [unwired: 2 in, 2 out]
            n200 = property on="What is this?" class="Bool (strict)"("Visible"=TRUE, "Caption.Text"=w356) -> ()  [unwired: 2 in, 2 out]
            n201 = property on="Rev/Fwd" class="Clust (strict)"("Visible"=FALSE) -> ()  [unwired: 2 in, 2 out]
          }
          frame "Camera" {
            n202 = call <vilib>:"Get Last Path Segment.vi"("String in"=w363) -> ("String out"=w364:string)  [unwired: 10 in]
            n203 = property on="What is this?" class="Bool (strict)"("Visible"=FALSE) -> ()  [unwired: 2 in, 2 out]
            n204 = property on="Motor" class="Clust (strict)"("Visible"=FALSE) -> ()  [unwired: 2 in, 2 out]
            n205 = property on="Rev/Fwd" class="Clust (strict)"("Visible"=FALSE) -> ()  [unwired: 2 in, 2 out]
            n206 = case shown="\"White Balance  **\"" w364 {
              tunnel: w363 -> [w370 w379 w388 w397 w406 _ w412]
              tunnel: w362 -> [w368 w376 w385 w394 w403 _ _]
              frame "Size  **" {
                n207 = Index Array(array=w368) -> (element=w367:cluster{string[]})  [unwired: 1 in]
                n208 = call <vilib>:"NT Read String.vi"("Name"=w370) -> ("String"=w369:string)  [unwired: 9 in, 1 out]
                n209 = Unbundle(w367) -> (w365:string[])
                n210 = Match First String(2:w365, 3:w369) -> (0:w366:i32)  [unwired: 1 out]
                n211 = property on="Ring" class="Ring (strict)"("Value"=w366, "Strings []"=w365) -> ()  [unwired: 2 in, 2 out]
                n212 = property on="Ring" class="Ring (strict)"("Visible"=TRUE) -> ()  [unwired: 2 in, 2 out]
                n213 = property on="Slider" class="Slide (strict)"("Visible"=FALSE) -> ()  [unwired: 2 in, 2 out]
              }
              frame "White Balance  **" {
                n214 = Index Array(array=w376, index=1) -> (element=w377:cluster{string[]})
                n215 = call <vilib>:"NT Read String.vi"("Name"=w379) -> ("String"=w378:string)  [unwired: 9 in, 1 out]
                n216 = Unbundle(w377) -> (w374:string[])
                n217 = Match First String(2:w374, 3:w378) -> (0:w373:i32)  [unwired: 1 out]
                n218 = property on="Ring" class="Ring (strict)"("Value"=w373, "Strings []"=w374) -> ()  [unwired: 2 in, 2 out]
                n219 = property on="Ring" class="Ring (strict)"("Visible"=TRUE) -> ()  [unwired: 2 in, 2 out]
                n220 = property on="Slider" class="Slide (strict)"("Visible"=FALSE) -> ()  [unwired: 2 in, 2 out]
              }
              frame "Exposure  **" {
                n221 = Index Array(array=w385, index=2) -> (element=w386:cluster{string[]})
                n222 = call <vilib>:"NT Read String.vi"("Name"=w388) -> ("String"=w387:string)  [unwired: 9 in, 1 out]
                n223 = Unbundle(w386) -> (w382:string[])
                n224 = Match First String(2:w382, 3:w387) -> (0:w383:i32)  [unwired: 1 out]
                n225 = property on="Ring" class="Ring (strict)"("Value"=w383, "Strings []"=w382) -> ()  [unwired: 2 in, 2 out]
                n226 = property on="Ring" class="Ring (strict)"("Visible"=TRUE) -> ()  [unwired: 2 in, 2 out]
                n227 = property on="Slider" class="Slide (strict)"("Visible"=FALSE) -> ()  [unwired: 2 in, 2 out]
              }
              frame "Exposure Priority  **" {
                n228 = Index Array(array=w394, index=3) -> (element=w395:cluster{string[]})
                n229 = call <vilib>:"NT Read String.vi"("Name"=w397) -> ("String"=w396:string)  [unwired: 9 in, 1 out]
                n230 = Unbundle(w395) -> (w391:string[])
                n231 = Match First String(2:w391, 3:w396) -> (0:w392:i32)  [unwired: 1 out]
                n232 = property on="Ring" class="Ring (strict)"("Value"=w392, "Strings []"=w391) -> ()  [unwired: 2 in, 2 out]
                n233 = property on="Ring" class="Ring (strict)"("Visible"=TRUE) -> ()  [unwired: 2 in, 2 out]
                n234 = property on="Slider" class="Slide (strict)"("Visible"=FALSE) -> ()  [unwired: 2 in, 2 out]
              }
              frame "Color Enable  **" {
                n235 = Index Array(array=w403, index=4) -> (element=w404:cluster{string[]})
                n236 = call <vilib>:"NT Read String.vi"("Name"=w406) -> ("String"=w405:string)  [unwired: 9 in, 1 out]
                n237 = Unbundle(w404) -> (w400:string[])
                n238 = Match First String(2:w400, 3:w405) -> (0:w401:i32)  [unwired: 1 out]
                n239 = property on="Ring" class="Ring (strict)"("Value"=w401, "Strings []"=w400) -> ()  [unwired: 2 in, 2 out]
                n240 = property on="Ring" class="Ring (strict)"("Visible"=TRUE) -> ()  [unwired: 2 in, 2 out]
                n241 = property on="Slider" class="Slide (strict)"("Visible"=FALSE) -> ()  [unwired: 2 in, 2 out]
              }
              frame Default {
                n242 = property on="Ring" class="Ring (strict)"("Visible"=FALSE) -> ()  [unwired: 2 in, 2 out]
                n243 = property on="Slider" class="Slide (strict)"("Visible"=FALSE) -> ()  [unwired: 2 in, 2 out]
              }
              frame "Brightness  **", "Color Level  **", "Compression  **", "FPS  **", "Sharpness  **" {
                n244 = call <vilib>:"NT Read Number.vi"("Name"=w412) -> ("Numeric"=w411:dbl)  [unwired: 9 in, 1 out]
                n245 = local write "Slider"(w411) -> ()
                n246 = property on="Slider" class="Slide (strict)"("Visible"=TRUE, "Scale.Maximum"=100.0 ("Scale.Range:Maximum")) -> ()  [unwired: 2 in, 2 out]
                n247 = property on="Ring" class="Ring (strict)"("Visible"=FALSE) -> ()  [unwired: 2 in, 2 out]
              }
            }
          }
        }
        n248 = property on="Progress" class="Clust (strict)"("Visible"=FALSE) -> ()  [unwired: 2 in, 2 out]
      }
      event "Test Name": Mouse Enter {
        # "Populate the ring with the list of tests"
        n249 = event-data() -> ()  [unwired: 1 in, 1 out]
        n250 = call <vilib>:"NT Read String Array.vi"("Name"="TestMode/TestList") -> ("String Array"=w419:string[])  [unwired: 9 in, 1 out]
        n251 = Build Array (concatenate)("Select the test to run...", w419) -> (w418:string[])
        n252 = property on="Test Name" class="Ring (strict)"("Strings []"=w418) -> ()  [unwired: 2 in, 2 out]
      }
      event "Test Name": Value Change {
        w421 = FALSE ("Visible")
        # "Tell the robot the test name to run"
        n253 = event-data() -> ("NewVal"=w425:u16)  [unwired: 1 in]
        n254 = property on="Test Name" class="Ring (strict)"() -> ("Strings []"=w426:string[])  [unwired: 2 in, 2 out]
        n255 = local write "Progress"(T4 {"Test Progress"=0, "Test Progress Text"=""} ("Progress")) -> ()
        n256 = Index Array(array=w426, index=w425) -> (element=w424:string)
        n257 = call <vilib>:"NT Write String.vi"("String"=w424, "Name"="TestMode/TestName") -> ()  [unwired: 9 in, 1 out]
        n258 = property on="Progress" class="Clust (strict)"("Visible"=TRUE) -> ()  [unwired: 2 in, 2 out]
        n259 = property on="Motor" class="Clust (strict)"("Visible"=w421) -> ()  [unwired: 2 in, 2 out]
        n260 = property on="Slider" class="Slide (strict)"("Visible"=w421) -> ()  [unwired: 2 in, 2 out]
        n261 = property on="What is this?" class="Bool (strict)"("Visible"=w421) -> ()  [unwired: 2 in, 2 out]
        n262 = property on="Rev/Fwd" class="Clust (strict)"("Visible"=w421) -> ()  [unwired: 2 in, 2 out]
        n263 = property on="Ring" class="Ring (strict)"("Visible"=w421) -> ()  [unwired: 2 in, 2 out]
      }
      event "Listbox": Double Click {
        n264 = event-data() -> ("PlatMods.Shift"=w429:bool, "Row"=w431:i32)  [unwired: 1 in]
        n265 = case shown="False" w429 {
          tunnel: w431 -> [w435 _]
          tunnel: 1 -> [w434 _]
          frame False {
            n266 = property on="Listbox" class="LstBox (strict)"() -> ("Item Symbols"=w433:i32[])  [unwired: 2 in, 2 out]
            n267 = Replace Array Subset(array=w433, new element=w434, index=w435) -> (w432:i32[])
            n268 = property on="Listbox" class="LstBox (strict)"("Item Symbols"=w432) -> ()  [unwired: 2 in, 2 out]
          }
          frame True {
            w436 = 0 ("Top Row")
            n269 = property on="Listbox" class="LstBox (strict)"() -> ("Number of Rows"=w438:u32)  [unwired: 2 in, 2 out]
            n270 = Initialize Array(0, w438) -> (w437:i32[])
            n271 = property on="Listbox" class="LstBox (strict)"("Top Row"=w436, "Value"=w436, "Item Symbols"=w437) -> ()  [unwired: 2 in, 2 out]
          }
        }
      }
      event "Listbox": Key Down {
        n272 = event-data() -> ("VKey"=w442:T17)  [unwired: 1 in]
        n273 = case shown="\"Left\", \"Right\"" w442 {
          selector: w442 -> [w447 _]
          tunnel: eventvkey."Left" ("VKey") -> [w445 _]
          frame "Left", "Right" {
            n274 = Equal?(x=w445, y=w447) -> (x = y?=w446:bool)
            n275 = Select(t=0, s=w446, f=1) -> (s? t:f=w448:i32)
            n276 = property on="Listbox" class="LstBox (strict)"() -> ("Item Symbols"=w451:i32[])  [unwired: 2 in, 2 out]
            n277 = Replace Array Subset(array=w451, new element=w448, index="Listbox") -> (w450:i32[])
            n278 = property on="Listbox" class="LstBox (strict)"("Item Symbols"=w450) -> ()  [unwired: 2 in, 2 out]
          }
          frame Default {
          }
        }
      }
      event "DB Camera Config": Value Change {
        n279 = event-data() -> ("NewVal"=w455:bool)  [unwired: 1 in]
        n280 = case shown="False" w455 {
          tunnel: w454 -> [w464 _]
          tunnel: [w457 w475] -> w453
          tunnel: w452 -> [w456 w475]
          frame False {
            w471 = "Camera"
            w474 = FALSE ("Visible")
            n281 = local read "Camera Settings"() -> (w463:T1)
            n282 = Index Array(array=w464) -> (element=w467:cluster{string[]})  [unwired: 1 in]
            n283 = Unbundle(w463) -> ("Frate Rate"=w462:i32, "Compression"=w461:i32, "Size"=w465:u16)
            n284 = Unbundle(w467) -> (w466:string[])
            n285 = Index Array(array=w466, index=w465) -> (element=w460:string)
            n286 = call-poly <vilib>:"Write Key.vi"("section"=w471, "value"=w460, "key"="Size", "refnum"=w456) -> ("refnum out"=w473:T15)  [unwired: 2 in, 5 out]
            n287 = call-poly <vilib>:"Write Key.vi"("section"=w471, "value"=w462, "key"="FrameRate", "refnum"=w473) -> ("refnum out"=w472:T15)  [unwired: 1 in, 6 out]
            n288 = property on="Camera Settings" class="Clust (strict)"("Visible"=w474) -> ()  [unwired: 2 in, 2 out]
            n289 = local write "DB Camera Config"(w474) -> ()
            n290 = call-poly <vilib>:"Write Key.vi"("section"=w471, "value"=w461, "key"="Compression", "refnum"=w472) -> ("refnum out"=w458:T15)  [unwired: 1 in, 6 out]
            n291 = call <vilib>:"Close Config Data.vi"("refnum"=w458) -> ("file path"=w459:path)  [unwired: 2 in, 8 out]
            n292 = call <vilib>:"Open Config Data.vi"("configuration file path"=w459) -> ("refnum"=w457:T15)  [unwired: 8 in, 2 out]
          }
          frame True {
            n293 = property on="Camera Settings" class="Clust (strict)"("Visible"=TRUE) -> ()  [unwired: 2 in, 2 out]
          }
        }
      }
      event "Camera Settings": Value Change {
        n294 = event-data() -> ("NewVal"=w488:T1)  [unwired: 1 in]
        n295 = Index Array(array=w484) -> (element=w483:cluster{string[]})  [unwired: 1 in]
        n296 = Unbundle(w488) -> ("Frate Rate"=w479:i32, "Compression"=w478:i32, "Size"=w481:u16)
        n297 = Unbundle(w483) -> (w482:string[])
        n298 = Index Array(array=w482, index=w481) -> (element=w480:string)
        n299 = Format Into String(format string="%s   %dfps   %d%%", w480, w479, w478) -> (resulting string=w485:string)  [unwired: 2 in, 1 out]
        n300 = Build Array(w485) -> (w486:string[])
        n301 = property on="DB Camera Config" class="Bool (strict)"("Strings [4]"=w486) -> ()  [unwired: 2 in, 2 out]
      }
      event "Motor.Enable": Value Change {
        n302 = event-data() -> ("NewVal"=w494:bool)  [unwired: 1 in]
        n303 = Unbundle("Motor") -> ("Value"=w493:dbl)  [unwired: 1 out]
        n304 = Select(t=w493, s=w494, f=0.0) -> (s? t:f=w491:dbl)
        n305 = call <vilib>:"NT Write Number.vi"("Numeric"=w491, "Name"=w490) -> ()  [unwired: 9 in, 1 out]
      }
      event "Slider": Value Change {
        n306 = event-data() -> ("NewVal"=w497:dbl)  [unwired: 1 in]
        n307 = call <vilib>:"NT Write Number.vi"("Numeric"=w497, "Name"=w498) -> ()  [unwired: 9 in, 1 out]
      }
      event "What is this?": Value Change {
        n308 = event-data() -> ("NewVal"=w502:bool)  [unwired: 1 in]
        n309 = Boolean To (0,1)(Boolean=w502) -> (0, 1=w501:i16)
        n310 = call <vilib>:"NT Write Number.vi"("Numeric"=w501, "Name"=w500) -> ()  [unwired: 9 in, 1 out]
      }
      event "Rev/Fwd": Value Change {
        n311 = event-data() -> ("NewVal.Forward"=w510:bool, "NewVal.Reverse"=w509:bool)  [unwired: 1 in]
        n312 = Boolean To (0,1)(Boolean=w510) -> (0, 1=w506:i16)
        n313 = Boolean To (0,1)(Boolean=w509) -> (0, 1=w508:i16)
        n314 = Negate(x=w508) -> (-x=w507:i16)
        n315 = Add(x=w506, y=w507) -> (x+y=w505:i16)
        n316 = call <vilib>:"NT Write Number.vi"("Numeric"=w505, "Name"=w504) -> ()  [unwired: 9 in, 1 out]
      }
      event "Ring": Value Change {
        n317 = event-data() -> ("NewVal"=w514:u16)  [unwired: 1 in]
        n318 = property on="Ring" class="Ring (strict)"() -> ("Strings []"=w515:string[])  [unwired: 2 in, 2 out]
        n319 = Index Array(array=w515, index=w514) -> (element=w513:string)
        n320 = call <vilib>:"NT Write String.vi"("String"=w513, "Name"=w512) -> ()  [unwired: 9 in, 1 out]
      }
    }
  }
  n321 = Index Array(array=w34) -> (element=w35:cluster{string[]})  [unwired: 1 in]
  n322 = Unbundle(w35) -> (w33:string[])
  n323 = call <vilib>:"Application Directory.vi"() -> ("Application Directory"=w1:path)
  n324 = Match First String(2:w33, 3:w32) -> (0:w31:i32)  [unwired: 1 out]
  n325 = while {
    tunnel: w1 -> [_]
    stop <- FALSE stop-if-true
    n326 = local read "Robot IP"() -> (w517:string)
    n327 = Wait (ms)(milliseconds to wait=u32 100) -> ()  [unwired: 1 out]
    n328 = case shown="True" "Transfer CSV to cRIO" {
      tunnel: "working directory" -> [_ w548]
      tunnel: w517 -> [_ w552]
      frame False {
      }
      frame True {
        w553 = ""
        w554 = "anonymous"
        w555 = "/2013AutoModesJava.csv"
        n329 = Build Path(base path=w548, name or relative path="2013AutoModesJavaLast.csv") -> (appended path=w551:path)
        n330 = call <vilib>:"FTP Get File.vi"("active (T)"=FALSE, "password"=w553, "binary (F)"=TRUE, "user"=w554, "local path"=w551, "remote path"=w555, "host"=w552) -> ("error out"=w545:errorcluster)  [unwired: 3 in, 1 out]
        n331 = case shown="No Error" w545 {
          tunnel: ["Saved Last" "Save Failed"] -> w544
          frame No Error {
          }
          frame Error {
          }
        }
        "standard output" <- w544
        n332 = Build Path(base path=w548, name or relative path="2013AutoModesJava.csv") -> (appended path=w550:path)
        n333 = call <vilib>:"FTP Put File.vi"("active (T)"=FALSE, "password"=w553, "binary (F)"=TRUE, "user"=w554, "error in (no error)"=w545, "local path"=w550, "remote path"=w555, "host"=w552) -> ("file error"=w547:errorcluster)  [unwired: 2 in, 1 out]
        n334 = case shown="Error" w547 {
          tunnel: ["Successfully Completed" "Transfer Failed"] -> w546
          frame No Error {
          }
          frame Error {
          }
        }
        n335 = local write "standard output"(w546) -> ()
      }
    }
    n336 = case shown="True" "Transfer INI From cRIO" {
      tunnel: "working directory" -> [_ w528]
      tunnel: w517 -> [_ w537]
      frame False {
      }
      frame True {
        n337 = Build Path(base path=w528, name or relative path="wpilib-preferences.ini") -> (appended path=w530:path)
        n338 = Build Path(base path=w528, name or relative path="wpilib-preferencesLast.ini") -> (appended path=w527:path)
        n339 = call <vilib>:"Check if File or Folder Exists.vi"("path"=w530) -> ("error out"=w532:errorcluster, "file or folder exists?"=w526:bool, "dup path"=w531:path)  [unwired: 8 in]
        n340 = Move(source path=w531, error in=w532, 9:w526, 10:w527) -> (error out=w525:errorcluster)  [unwired: 1 in, 2 out]
        n341 = case shown="No Error" w525 {
          tunnel: ["/nSaved Last" "/nSave Failed"] -> w524
          frame No Error {
          }
          frame Error {
          }
        }
        n342 = call <vilib>:"FTP Get File.vi"("active (T)"=FALSE, "password"="", "binary (F)"=TRUE, "user"="anonymous", "error in (no error)"=w525, "local path"=w530, "remote path"="/wpilib-preferences.ini", "host"=w537) -> ("error out"=w522:errorcluster)  [unwired: 2 in, 1 out]
        n343 = local write "standard output"(w524) -> ()
        n344 = case shown="Error" w522 {
          tunnel: ["Successfully Completed" "/nTransfer Failed"] -> w523
          frame No Error {
          }
          frame Error {
          }
        }
        n345 = local write "standard output"(w523) -> ()
      }
    }
  }
  n346 = flat-sequence {
    frame #0 {
      # "Autonomous Mode Script Select"
      n347 = control-ref of="Autonomous Mode"() -> (w566:refnum<vi>)
      n348 = call "DashboardSelectAuto.vi"("Table Prefix"="Autonomous mode", "Autonomous Mode Ring"=w566) -> ()  [unwired: 9 in]
    }
  }
  n349 = local write "working directory"(w1) -> ()
  n350 = Bundle("value"=w37, "value"=w36, "index"=w31) -> (w25:cluster{"value":i32, "value":i32, "index":i32})  [unwired: 1 out]
  n351 = property on="What is this?" class="Bool (strict)"("Visible"=w48) -> ()  [unwired: 2 in, 2 out]
  n352 = property on="Motor" class="Clust (strict)"("Visible"=w48) -> ()  [unwired: 2 in, 2 out]
  n353 = property on="Progress" class="Clust (strict)"("Visible"=w48) -> ()  [unwired: 2 in, 2 out]
  n354 = property on="Ring" class="Ring (strict)"("Visible"=w48) -> ()  [unwired: 2 in, 2 out]
  n355 = property on="Camera Settings" class="Clust (strict)"("Val(Sgnl)"=w25) -> ()  [unwired: 2 in, 2 out]
  n356 = property on="Rev/Fwd" class="Clust (strict)"("Visible"=w48) -> ()  [unwired: 2 in, 2 out]
  n357 = local write "DB Camera Config"(w48) -> ()
  n358 = property on="Camera Settings" class="Clust (strict)"("Visible"=w48) -> ()  [unwired: 2 in, 2 out]
  n359 = disable-structure shown="Disabled" {
    frame Disabled {
      n360 = call "BB_Check_Camera_IP_Change.vi"() -> ()  [unwired: 11 in, 1 out]
    }
    frame Enabled {
    }
  }
